vi "Convert_Temp.vi"() -> ()   [LabVIEW 2022 SP3]
panel:
  out "Tf":dbl format="%#_13g"
  out "Tc":dbl format="%#_13g"
  in  "Tk":dbl format="%#_13g"
  # "Convert_Temperature:\nEnter any temperature in Kelvin to see it in both Fahrenheit and Celsius."
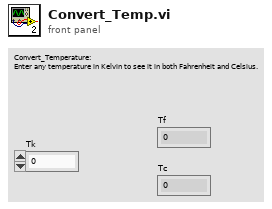
[diagram p1: front panel]
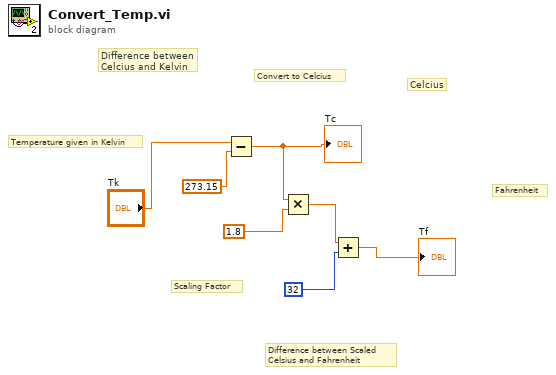
[diagram p0: block diagram]
diagram:
  # "Difference between \nCelcius and Kelvin"
  # "Difference between Scaled\nCelsius and Fahrenheit"
  # "Scaling Factor"
  # "Fahrenheit"
  # "Celcius"
  # "Convert to Celcius"
  # "Temperature given in Kelvin"
  n1 = Subtract(x="Tk", y=273.15) -> (x-y=w5:dbl)
  "Tc" <- w5
  n2 = Multiply(x=w5, y=1.8) -> (x*y=w2:dbl)
  n3 = Add(x=w2, y=32) -> (x+y=→"Tf":dbl)
